vi "Generic command handler.vi"(8 "error in (no error)":errorcluster, 10 "Message in":refnum<class "GenericMessage.lvclass">, 11 "DAQMH121119OrcaFlash in":refnum<class "DAQOrcaFlash.lvclass">) -> (0 "error out":errorcluster, 2 "value":string, 3 "DAQMH121119OrcaFlash out":refnum<class "DAQOrcaFlash.lvclass">)   [LabVIEW 2012, in "DAQOrcaFlash.lvclass"]
doc: "The generic_command_handler processes the command 'generic'. Commands which are not part of the predefined list of commands fall under the 'generic' command for special activity."
uses:
  DAQOrcaFlash.lvclass
  <vilib>/Distrio/Murmex/GenericMessage/GenericMessage.lvclass
  <vilib>/Distrio/Murmex/Murmex/Murmex.lvclass
  <vilib>/Distrio/Murmex/Message/Message.lvclass
panel:
  # "This method is called when the GENERIC\ntrigger is sent. \n\nOverride this method when your component needs to\nrespond to this trigger. \n\nCall parent for proper implementation"
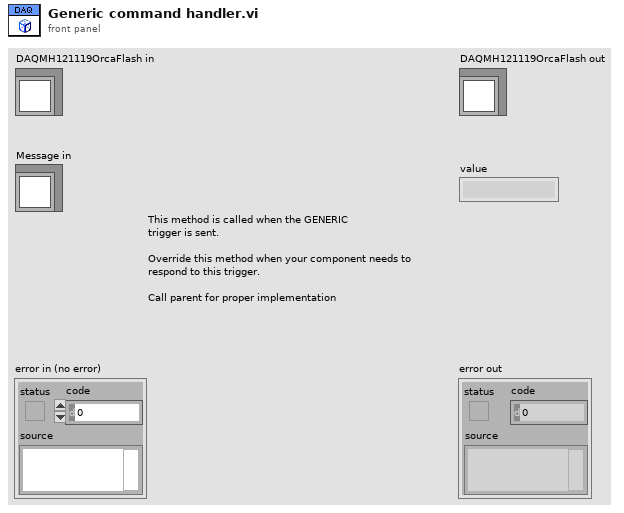
[diagram p1: front panel]
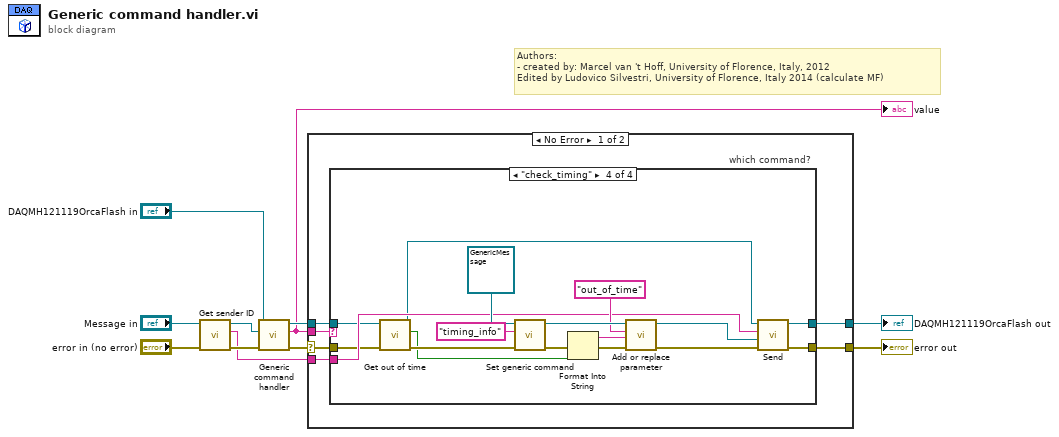
[diagram p0: block diagram]
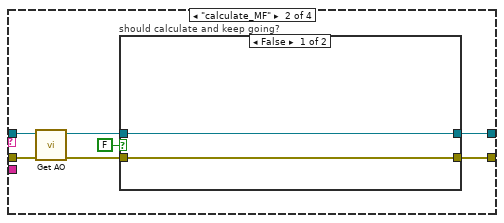
[diagram p3: hidden frame]
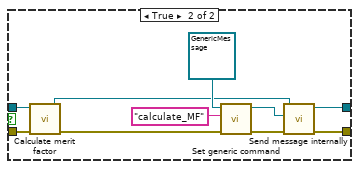
[diagram p4: hidden frame]
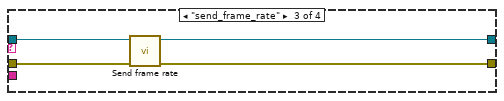
[diagram p5: hidden frame]
diagram:
  # "Authors: \n- created by: Marcel van 't Hoff, University of Florence, Italy, 2012\nEdited by Ludovico Silvestri, University of Florence, Italy 2014 (calculate MF)"
  n1 = call <vilib>:"Get sender ID.vi"("error in (no error)"="error in (no error)", "Message in"="Message in") -> ("error out"=w4:errorcluster, "sender"=w1:string, "Message out"=w2:refnum<class "GenericMessage.lvclass">)  [unwired: 7 in]
  n2 = call-parent "Generic command handler.vi"("error in (no error)"=w4, "Message in"=w2, "Murmex in"="DAQMH121119OrcaFlash in") -> ("error out"=w9:errorcluster, "value"=w5:string, "Murmex out"=w6:refnum<class "DAQOrcaFlash.lvclass">)  [unwired: 6 in]
  "value" <- w5
  n3 = case shown="No Error" w9 {
    selector: w9 -> [w16 w61]
    tunnel: [w15 w61] -> w8
    tunnel: [w14 w60] -> w7
    tunnel: w6 -> [w13 w60]
    tunnel: w5 -> [w17 _]
    tunnel: w1 -> [w12 _]
    frame No Error {
      n4 = case "which command?" shown="\"check_timing\"" w17 {
        tunnel: w16 -> [w19 w26 w42 w48]
        tunnel: w13 -> [w18 w25 w41 w46]
        tunnel: [w19 w22 w40 w50] -> w15
        tunnel: [w18 w21 w39 w43] -> w14
        tunnel: w12 -> [_ _ _ w49]
        frame Default {
        }
        frame "calculate_MF" {
          n5 = call-dynamic "Get AO.vi"("error in (no error)"=w26, "DAQOrcaFlash in"=w25) -> ("error out"=w24:errorcluster, "DAQOrcaFlash out"=w23:refnum<class "DAQOrcaFlash.lvclass">)  [unwired: 7 in, 1 out]
          n6 = case "should calculate and keep going?" shown="False" FALSE {
            tunnel: w24 -> [w28 w38]
            tunnel: w23 -> [w27 w37]
            tunnel: [w28 w32] -> w22
            tunnel: [w27 w34] -> w21
            frame False {
            }
            frame True {
              n7 = call-dynamic "Calculate merit factor.vi"("error in (no error)"=w38, "DAQOrcaFlash in"=w37) -> ("error out"=w29:errorcluster, "DAQOrcaFlash out"=w30:refnum<class "DAQOrcaFlash.lvclass">)  [unwired: 8 in]
              n8 = call <vilib>:"Set generic command.vi"("error in (no error)"=w29, "generic command"="calculate_MF", "GenericMessage in"=refnum<class "GenericMessage.lvclass"> refnum ("GenericMessage")) -> ("error out"=w33:errorcluster, "GenericMessage out"=w31:refnum<class "GenericMessage.lvclass">)  [unwired: 7 in]
              n9 = call <vilib>:"Send message internally.vi"("error in (no error)"=w33, "Message"=w31, "Murmex in"=w30) -> ("error out"=w32:errorcluster, "Murmex out"=w34:refnum<class "DAQOrcaFlash.lvclass">)  [unwired: 7 in]
            }
          }
        }
        frame "send_frame_rate" {
          n10 = call-dynamic "Send frame rate.vi"("error in (no error)"=w42, "DAQOrcaFlash in"=w41) -> ("error out"=w40:errorcluster, "DAQOrcaFlash out"=w39:refnum<class "DAQOrcaFlash.lvclass">)  [unwired: 8 in]
        }
        frame "check_timing" {
          n11 = call-dynamic "Get out of time.vi"("error in (no error)"=w48, "DAQOrcaFlash in"=w46) -> ("error out"=w47:errorcluster, "out of time?"=w44:bool, "DAQOrcaFlash out"=w45:refnum<class "DAQOrcaFlash.lvclass">)  [unwired: 7 in]
          n12 = call <vilib>:"Set generic command.vi"("error in (no error)"=w47, "generic command"="timing_info", "GenericMessage in"=refnum<class "GenericMessage.lvclass"> refnum ("Distrio Murmex 1.5:GenericMessage")) -> ("error out"=w53:errorcluster, "GenericMessage out"=w55:refnum<class "GenericMessage.lvclass">)  [unwired: 7 in]
          n13 = Format Into String(error in=w53, w44) -> (resulting string=w51:string, error out=w52:errorcluster)  [unwired: 2 in]
          n14 = call <vilib>:"Add or replace parameter.vi"("error in (no error)"=w52, "value"=w51, "name"="out_of_time", "Message in"=w55) -> ("error out"=w57:errorcluster, "Message out"=w56:refnum<class "GenericMessage.lvclass">)  [unwired: 6 in]
          n15 = call <vilib>:"Send.vi"("error in (no error)"=w57, "Message"=w56, "recipient"=w49, "Murmex in"=w45) -> ("error out"=w50:errorcluster, "Murmex out"=w43:refnum<class "DAQOrcaFlash.lvclass">)  [unwired: 6 in]
        }
      }
    }
    frame Error {
    }
  }
  "error out" <- w8
  "DAQMH121119OrcaFlash out" <- w7
